vi "getCalculationSolution.vi"(10 "calculationResult":dbl, 11 "View.lvclass":refnum<class "View.lvclass">) -> (3 "View out":refnum<class "View.lvclass">)   [LabVIEW 2016, in "View.lvclass"]
uses:
  View.lvclass
  View.lvclass/View.ctl
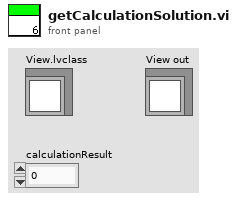
[diagram p1: front panel]
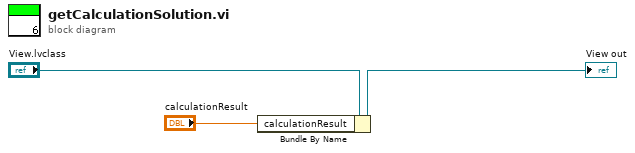
[diagram p0: block diagram]
diagram:
  n1 = Bundle By Name(cluster="View.lvclass", "calculationResult"="calculationResult") -> (→"View out":refnum<class "View.lvclass">)
